vi "ObjectFactory.vi"(0 "GOject":refnum<vi>, 5 "error in (no error)":errorcluster) -> (14 "Object":refnum<class "Object.lvclass">, 15 "Is Indicator":bool, 16 "Is Control":bool, 17 "Is Visible":bool, 19 "error out":errorcluster)   [LabVIEW 2014, in "FrontPanelPublisher.lvlib" / "WebFrontPanel.lvclass"]
doc: "Convert FP refs into \"HTML\" objects"
uses:
  WebFrontPanel.lvclass
  Object_class/Object.lvclass
  Object_class/Attributes.ctl
  Object_class/Coordinates.ctl
  Control_class/Attributes.ctl
  Text_class/Text.lvclass
  BooleanControl_class/Attributes.ctl
  Numeric_class/Attributes.ctl
  String_class/Attributes.ctl
  Graph_class/Attributes.ctl
  Select_class/Attributes.ctl
  Progressbar_class/Attributes.ctl
  Text_class/Attributes.ctl
  Control_class/Control.lvclass
  BooleanControl_class/BooleanControl.lvclass
  Graph_class/Graph.lvclass
  Numeric_class/Numeric.lvclass
  FrontPanelPublisher.lvlib
  String_class/String.lvclass
  Select_class/Select.lvclass
  Progressbar_class/Progressbar.lvclass
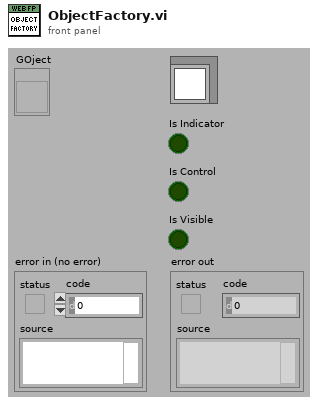
[diagram p1: front panel]
types:
  T1 = typedef "FrontPanelPublisher.lvlib/Object.lvclass/Attributes.ctl" = cluster{"UID":i32, "Type":string, "Coordinates":T2, "Reference":refnum<vi>}
  T2 = typedef "FrontPanelPublisher.lvlib/Object.lvclass/Coordinates.ctl" = cluster{"Left":i32, "Top":i32, "Height":u32, "Width":u32}
  T3 = typedef "FrontPanelPublisher.lvlib/Control.lvclass/Attributes.ctl" = cluster{"Description":string, "Indicator":bool, "Default Value":variant, "Control Index":i32, "Label":refnum<class "Text.lvclass">, "Caption":refnum<class "Text.lvclass">, "Use Picture":bool, "Image1 b64":string, "Image2 b64":string}
  T4 = typedef "FrontPanelPublisher.lvlib/BooleanControl.lvclass/Attributes.ctl" = cluster{"Boolean ref":refnum<vi>, "Switching":bool, "Boolean Strings":string[], "Text":refnum<class "Text.lvclass">}
  T5 = typedef "FrontPanelPublisher.lvlib/Numeric.lvclass/Attributes.ctl" = cluster{"unused":dbl}
  T6 = typedef "FrontPanelPublisher.lvlib/String.lvclass/Attributes.ctl" = cluster{"unused":string}
  T7 = typedef "FrontPanelPublisher.lvlib/Graph.lvclass/Attributes.ctl" = cluster{"not used":dbl}
  T8 = typedef "FrontPanelPublisher.lvlib/Select.lvclass/Attributes.ctl" = cluster{"not used":dbl}
  T9 = typedef "FrontPanelPublisher.lvlib/Progressbar.lvclass/Attributes.ctl" = cluster{"not used":dbl}
  T10 = cluster{"Object":T1, "Control":T3, "Boolean":T4, "Numeric":T5, "String":T6, "Graph":T7, "Select":T8, "Progressbar":T9, "Object out":refnum<class "Object.lvclass">, "Label":refnum<class "Text.lvclass">, "Caption":refnum<class "Text.lvclass">, "Is Indicator":bool, "Is Control":bool, "Is Visible":bool}
  T11 = typedef "FrontPanelPublisher.lvlib/Text.lvclass/Attributes.ctl" = cluster{"Text":string, "Font":string, "Font Size":u32, "Visible":bool}
  T12 = typedef "LVRectTypeDef.ctl" = cluster{"Left":i16, "Top":i16, "Right":i16, "Bottom":i16}
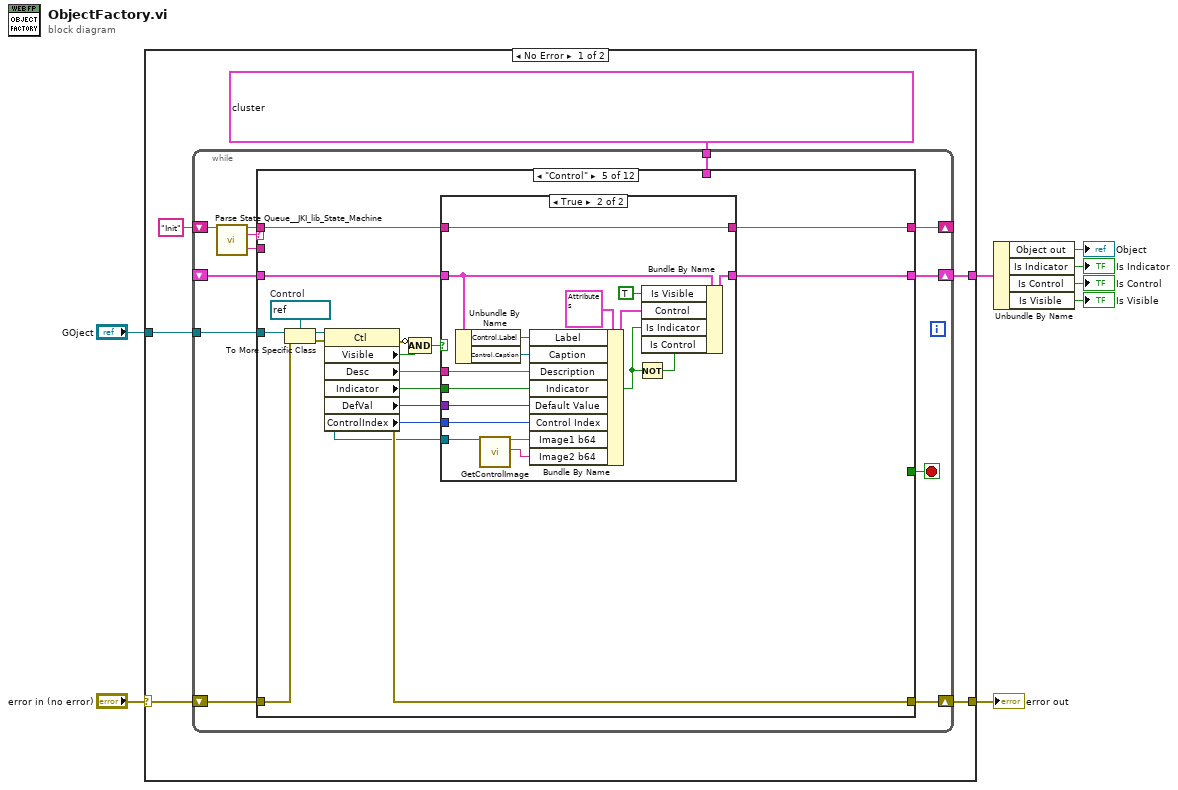
[diagram p0: block diagram]
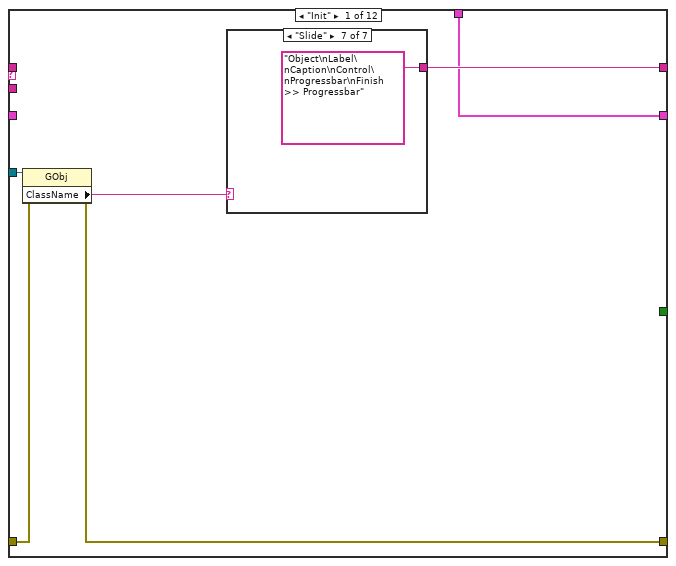
[diagram p2: hidden frame]
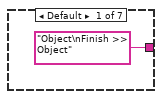
[diagram p3: hidden frame]
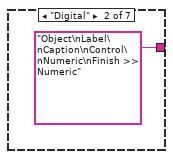
[diagram p4: hidden frame]
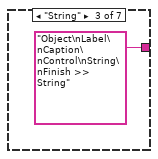
[diagram p5: hidden frame]
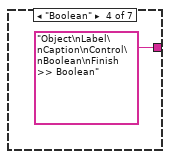
[diagram p6: hidden frame]
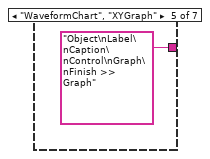
[diagram p7: hidden frame]
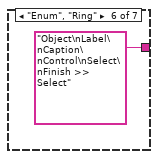
[diagram p8: hidden frame]
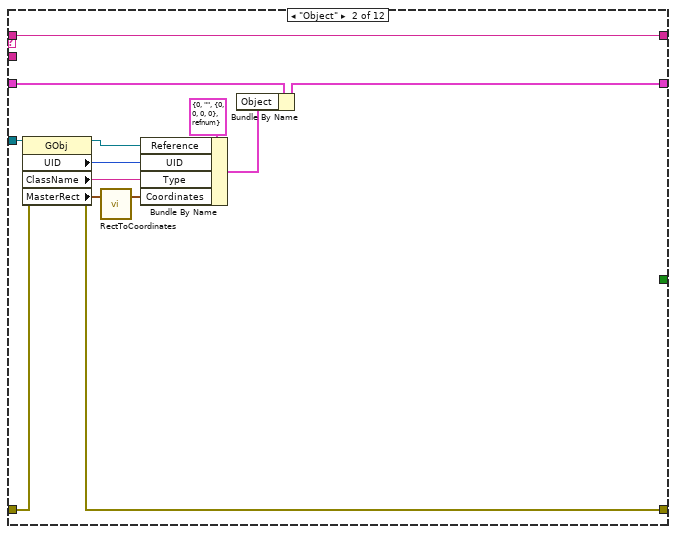
[diagram p9: hidden frame]
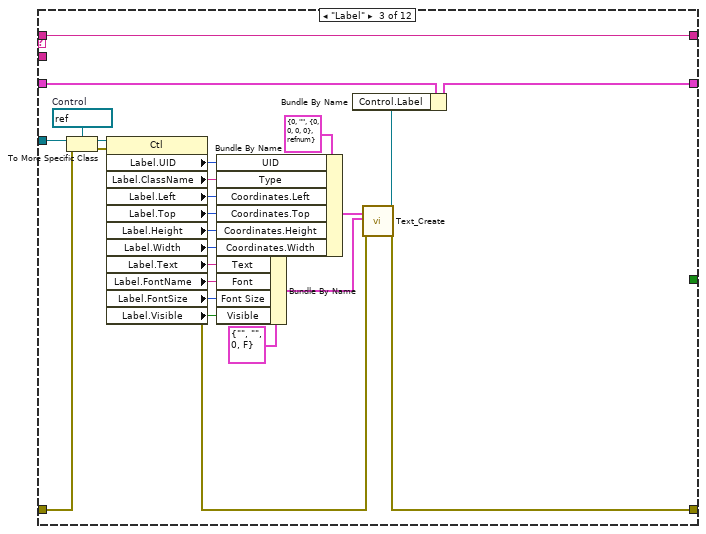
[diagram p10: hidden frame]
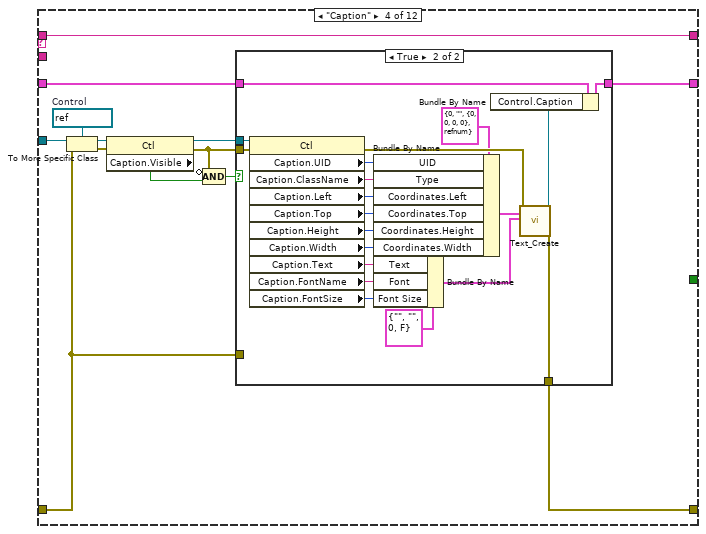
[diagram p11: hidden frame]
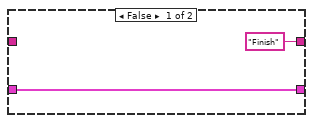
[diagram p13: hidden frame]
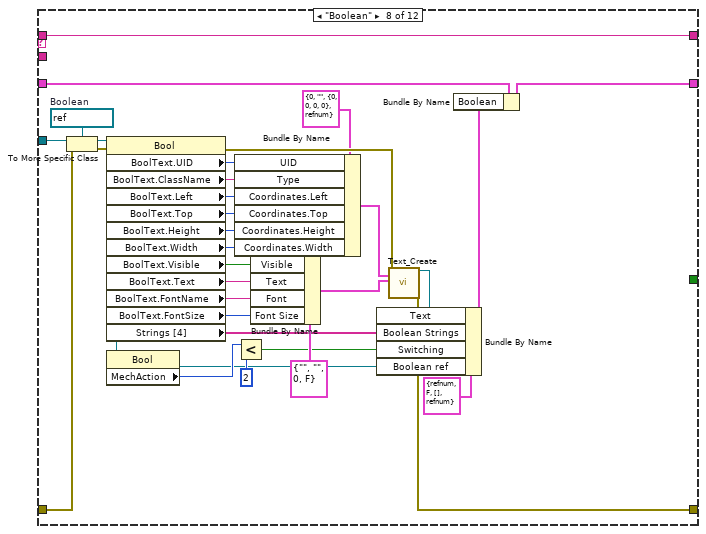
[diagram p16: hidden frame]
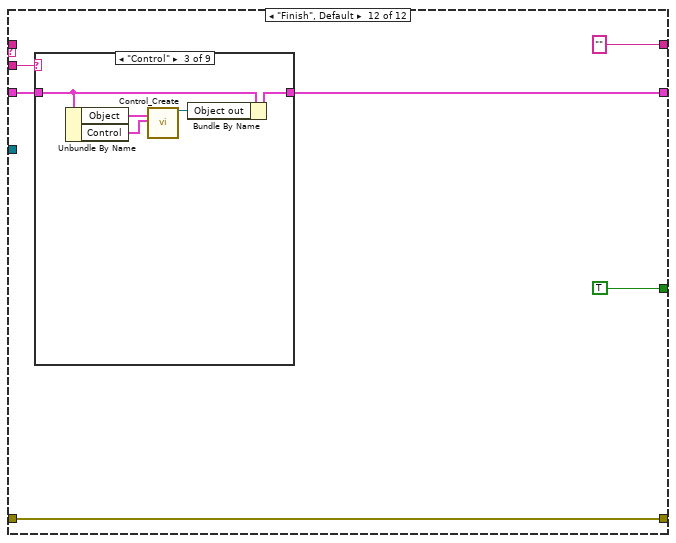
[diagram p20: hidden frame]
diagram:
  n1 = case shown="No Error" "error in (no error)" {
    selector: "error in (no error)" -> [w13 w245]
    tunnel: [w14 w245] -> w7
    tunnel: "GOject" -> [w12 _]
    tunnel: [w9 _] -> w5
    frame No Error {
      n2 = while {
        tunnel: w12 -> [w24]
        shift-right: [w15] -> _
        shift-left: "Init" -> [w19]
        shift-right: [w23] -> w9
        shift-left: _ -> [w22]
        shift-right: [w25] -> w14
        shift-left: w13 -> [w26]
        tunnel: T10 {"Object"={"UID"=0, "Type"="", "Coordinates"={"Left"=0, "Top"=0, "Height"=0, "Width"=0}, "Reference"=refnum}, "Control"={"Description"="", "Indicator"=FALSE, "Default Value"=variant, "Control Index"=0, "Label"=refnum, "Caption"=refnum, "Use Picture"=FALSE, "Image1 b64"="", "Image2 b64"=""}, "Boolean"={"Boolean ref"=refnum, "Switching"=FALSE, "Boolean Strings"=[], "Text"=refnum}, "Numeric"={"unused"=0.0}, "String"={"unused"=""}, "Graph"={"not used"=0.0}, "Select"={"not used"=0.0}, "Progressbar"={"not used"=0.0}, "Object out"=refnum, "Label"=refnum, "Caption"=refnum, "Is Indicator"=FALSE, "Is Control"=FALSE, "Is Visible"=FALSE} -> [w21]
        stop <- w20 stop-if-true
        n3 = call <vilib>:"Parse State Queue__JKI_lib_State_Machine.vi"("State Queue"=w19) -> ("Remaining States"=w16:string, "Current State"=w18:string, "Arguments"=w17:string)  [unwired: 12 in]
        n4 = case shown="\"Control\"" w18 {
          tunnel: w24 -> [w30 w48 w72 w84 w124 _ _ w180 _ _ _ _]
          tunnel: [w28 w45 w60 w79 w115 w149 w152 w177 w186 w189 w192 ""] -> w15
          tunnel: [w27 w47 w61 w80 w118 w148 w151 w178 w184 w187 w190 w194] -> w23
          tunnel: w22 -> [_ w46 w62 w81 w123 w148 w151 w179 w184 w187 w190 w193]
          tunnel: [w31 w51 w75 w88 w126 w147 w150 w183 w185 w188 w191 w198] -> w25
          tunnel: w26 -> [w32 w52 w76 w87 w127 w147 w150 w182 w185 w188 w191 w198]
          tunnel: w21 -> [w27 _ _ _ _ _ _ _ _ _ _ _]
          tunnel: [_ _ _ _ _ _ _ _ _ _ _ TRUE] -> w20
          tunnel: w17 -> [_ _ _ _ _ _ _ _ _ _ _ w195]
          tunnel: w16 -> [_ w45 w60 w79 w114 w149 w152 w177 w186 w189 w192 _]
          frame "Init" {
            n5 = property class="GObj"(reference=w30, error in=w32) -> (error out=w31:errorcluster, "ClassName"=w29:string)  [unwired: 1 out]
            n6 = case shown="\"Slide\"" w29 {
              tunnel: ["Object\nFinish >> Object" "Object\nLabel\nCaption\nControl\nNumeric\nFinish >> Numeric" "Object\nLabel\nCaption\nControl\nString\nFinish >> String" "Object\nLabel\nCaption\nControl\nBoolean\nFinish >> Boolean" "Object\nLabel\nCaption\nControl\nGraph\nFinish >> Graph" "Object\nLabel\nCaption\nControl\nSelect\nFinish >> Select" "Object\nLabel\nCaption\nControl\nProgressbar\nFinish >> Progressbar"] -> w28
              frame Default {
              }
              frame "Digital" {
              }
              frame "String" {
              }
              frame "Boolean" {
              }
              frame "WaveformChart", "XYGraph" {
              }
              frame "Enum", "Ring" {
              }
              frame "Slide" {
              }
            }
          }
          frame "Object" {
            n7 = property class="GObj"(reference=w48, error in=w52) -> (reference out=w40:refnum<vi>, error out=w51:errorcluster, "UID"=w49:i32, "ClassName"=w50:string, "MasterRect"=w42:T12)
            n8 = call "RectToCoordinates.vi"("Rect"=w42) -> ("Coordinates"=w41:T2)  [unwired: 2 in]
            n9 = Bundle By Name(cluster=T1 {"UID"=0, "Type"="", "Coordinates"={"Left"=0, "Top"=0, "Height"=0, "Width"=0}, "Reference"=refnum} ("Object Attributes"), "Reference"=w40, "UID"=w49, "Type"=w50, "Coordinates"=w41) -> (w43:T1)
            n10 = Bundle By Name(cluster=w46, "Object"=w43) -> (w47:T10)
          }
          frame "Label" {
            w74 = refnum<vi> refnum  # Control
            n11 = To More Specific Class(target class=w74, reference=w72, error in=w76) -> (specific class reference=w73:refnum<vi>, error out=w77:errorcluster)
            n12 = property class="Ctl"(reference=w73, error in=w77) -> (error out=w54:errorcluster, "Label.UID"=w71:i32, "Label.ClassName"=w70:string, "Label.Left"=w69:i32, "Label.Top"=w68:i32, "Label.Height"=w67:u32, "Label.Width"=w66:u32, "Label.Text"=w65:string, "Label.FontName"=w64:string, "Label.FontSize"=w63:u32, "Label.Visible"=w53:bool)  [unwired: 1 out]
            n13 = Bundle By Name(cluster=T1 {"UID"=0, "Type"="", "Coordinates"={"Left"=0, "Top"=0, "Height"=0, "Width"=0}, "Reference"=refnum} ("Object Attributes"), "UID"=w71, "Type"=w70, "Coordinates.Left"=w69, "Coordinates.Top"=w68, "Coordinates.Height"=w67, "Coordinates.Width"=w66) -> (w57:T1)
            n14 = Bundle By Name(cluster=T11 {"Text"="", "Font"="", "Font Size"=0, "Visible"=FALSE} ("Text Attributes"), "Text"=w65, "Font"=w64, "Font Size"=w63, "Visible"=w53) -> (w56:T11)
            n15 = call "Text_Create.vi"("Object Attributes"=w57, "Text Attributes"=w56, "error in (no error)"=w54) -> ("reference out"=w55:refnum<class "Text.lvclass">, "error out"=w75:errorcluster)  [unwired: 15 in]
            n16 = Bundle By Name(cluster=w62, "Control.Label"=w55) -> (w61:T10)
          }
          frame "Caption" {
            w86 = refnum<vi> refnum  # Control
            n17 = To More Specific Class(target class=w86, reference=w84, error in=w87) -> (specific class reference=w85:refnum<vi>, error out=w90:errorcluster)
            n18 = property class="Ctl"(reference=w85, error in=w90) -> (reference out=w78:refnum<vi>, error out=w89:errorcluster, "Caption.Visible"=w83:bool)
            n19 = Compound Arithmetic op=AND(invert w89, w83) -> (w82:bool)
            n20 = case shown="True" w82 {
              tunnel: w81 -> [w91 w105]
              tunnel: [w91 w104] -> w80
              tunnel: w78 -> [_ w102]
              tunnel: w89 -> [_ w112]
              tunnel: [w92 w110] -> w88
              tunnel: w87 -> [w92 _]
              frame False {
              }
              frame True {
                n21 = property class="Ctl"(reference=w102, error in=w112) -> (error out=w111:errorcluster, "Caption.UID"=w101:i32, "Caption.ClassName"=w100:string, "Caption.Left"=w99:i32, "Caption.Top"=w98:i32, "Caption.Height"=w97:u32, "Caption.Width"=w96:u32, "Caption.Text"=w95:string, "Caption.FontName"=w94:string, "Caption.FontSize"=w93:u32)  [unwired: 1 out]
                n22 = Bundle By Name(cluster=T1 {"UID"=0, "Type"="", "Coordinates"={"Left"=0, "Top"=0, "Height"=0, "Width"=0}, "Reference"=refnum} ("Object Attributes"), "UID"=w101, "Type"=w100, "Coordinates.Left"=w99, "Coordinates.Top"=w98, "Coordinates.Height"=w97, "Coordinates.Width"=w96) -> (w107:T1)
                n23 = Bundle By Name(cluster=T11 {"Text"="", "Font"="", "Font Size"=0, "Visible"=FALSE} ("Text Attributes"), "Text"=w95, "Font"=w94, "Font Size"=w93) -> (w106:T11)
                n24 = call "Text_Create.vi"("Object Attributes"=w107, "Text Attributes"=w106, "error in (no error)"=w111) -> ("reference out"=w103:refnum<class "Text.lvclass">, "error out"=w110:errorcluster)  [unwired: 15 in]
                n25 = Bundle By Name(cluster=w105, "Control.Caption"=w103) -> (w104:T10)
              }
            }
          }
          frame "Control" {
            w125 = refnum<vi> refnum  # Control
            n26 = To More Specific Class(target class=w125, reference=w124, error in=w127) -> (specific class reference=w113:refnum<vi>, error out=w128:errorcluster)
            n27 = property class="Ctl"(reference=w113, error in=w128) -> (error out=w126:errorcluster, "Visible"=w116:bool, "Desc"=w122:string, "Indicator"=w121:bool, "DefVal"=w120:variant, "ControlIndex"=w119:i32)  [unwired: 1 out]
            n28 = Compound Arithmetic op=AND(invert w126, w116) -> (w117:bool)
            n29 = case shown="True" w117 {
              tunnel: w123 -> [w130 w140]
              tunnel: w122 -> [_ w146]
              tunnel: w121 -> [_ w136]
              tunnel: w120 -> [_ w145]
              tunnel: w119 -> [_ w144]
              tunnel: [w130 w131] -> w118
              tunnel: ["Finish" w141] -> w115
              tunnel: w114 -> [_ w141]
              tunnel: w113 -> [_ w132]
              frame False {
              }
              frame True {
                n30 = Unbundle By Name(w140) -> ("Control.Label"=w139:refnum<class "Text.lvclass">, "Control.Caption"=w138:refnum<class "Text.lvclass">)
                n31 = call "GetControlImage.vi"("Control ref"=w132) -> ("base64 encoded <img> string 1"=w134:string, "base64 encoded <img> string 2"=w133:string)  [unwired: 16 in, 1 out]
                n32 = Bundle By Name(cluster=T3 {"Description"="", "Indicator"=FALSE, "Default Value"=variant, "Control Index"=0, "Label"=refnum, "Caption"=refnum, "Use Picture"=FALSE, "Image1 b64"="", "Image2 b64"=""} ("Control Attributes"), "Label"=w139, "Caption"=w138, "Description"=w146, "Indicator"=w136, "Default Value"=w145, "Control Index"=w144, "Image1 b64"=w134, "Image2 b64"=w133) -> (w142:T3)
                n33 = Not(x=w136) -> (.not. x?=w135:bool)
                n34 = Bundle By Name(cluster=w140, "Is Visible"=TRUE, "Control"=w142, "Is Indicator"=w136, "Is Control"=w135) -> (w131:T10)
              }
            }
          }
          frame "Numeric" {
            # "All properties are queried at run time"
          }
          frame "String" {
            # "All properties are queried at run time"
          }
          frame "Boolean" {
            w181 = refnum<vi> refnum  # Boolean
            n35 = To More Specific Class(target class=w181, reference=w180, error in=w182) -> (specific class reference=w153:refnum<vi>, error out=w155:errorcluster)
            n36 = property class="Bool"(reference=w153, error in=w155) -> (error out=w176:errorcluster, "BoolText.UID"=w166:i32, "BoolText.ClassName"=w165:string, "BoolText.Left"=w164:i32, "BoolText.Top"=w163:i32, "BoolText.Height"=w162:u32, "BoolText.Width"=w161:u32, "BoolText.Visible"=w156:bool, "BoolText.Text"=w160:string, "BoolText.FontName"=w159:string, "BoolText.FontSize"=w158:u32, "Strings [4]"=w157:string[])  [unwired: 1 out]
            n37 = property class="Bool"(reference=w153) -> ("MechAction"=w154:u32)  [unwired: 1 in, 2 out]
            n38 = Bundle By Name(cluster=T1 {"UID"=0, "Type"="", "Coordinates"={"Left"=0, "Top"=0, "Height"=0, "Width"=0}, "Reference"=refnum} ("Object Attributes"), "UID"=w166, "Type"=w165, "Coordinates.Left"=w164, "Coordinates.Top"=w163, "Coordinates.Height"=w162, "Coordinates.Width"=w161) -> (w171:T1)
            n39 = Less?(x=w154, y=u32 2) -> (x < y?=w167:bool)
            n40 = Bundle By Name(cluster=T11 {"Text"="", "Font"="", "Font Size"=0, "Visible"=FALSE} ("Text Attributes"), "Visible"=w156, "Text"=w160, "Font"=w159, "Font Size"=w158) -> (w170:T11)
            n41 = call "Text_Create.vi"("Object Attributes"=w171, "Text Attributes"=w170, "error in (no error)"=w176) -> ("reference out"=w169:refnum<class "Text.lvclass">, "error out"=w183:errorcluster)  [unwired: 15 in]
            n42 = Bundle By Name(cluster=T4 {"Boolean ref"=refnum, "Switching"=FALSE, "Boolean Strings"=[], "Text"=refnum} ("BooleanControl Attributes"), "Text"=w169, "Boolean Strings"=w157, "Switching"=w167, "Boolean ref"=w153) -> (w168:T4)
            n43 = Bundle By Name(cluster=w179, "Boolean"=w168) -> (w178:T10)
          }
          frame "Graph" {
            # "All properties are queried at run time"
          }
          frame "Select" {
            # "All properties are queried at run time"
          }
          frame "Progressbar" {
            # "All properties are queried at run time"
          }
          frame "Finish", Default {
            n44 = case shown="\"Control\"" w195 {
              tunnel: [w199 w201 w207 w210 w218 w224 w230 w236 w242] -> w194
              tunnel: w193 -> [w199 w203 w208 w214 w220 w226 w232 w238 w244]
              frame Default {
              }
              frame "Object" {
                n45 = Unbundle By Name(w203) -> ("Object"=w202:T1)
                n46 = call "Object_Create.vi"("Object Attributes"=w202) -> ("reference out"=w200:refnum<class "Object.lvclass">)  [unwired: 17 in, 1 out]
                n47 = Bundle By Name(cluster=w203, "Object out"=w200) -> (w201:T10)
              }
              frame "Control" {
                n48 = Unbundle By Name(w208) -> ("Object"=w205:T1, "Control"=w204:T3)
                n49 = call "Control_Create.vi"("Object Attributes"=w205, "Control Attributes"=w204) -> ("reference out"=w206:refnum<class "Control.lvclass">)  [unwired: 16 in, 1 out]
                n50 = Bundle By Name(cluster=w208, "Object out"=w206) -> (w207:T10)
              }
              frame "Boolean" {
                n51 = Unbundle By Name(w214) -> ("Object"=w213:T1, "Control"=w212:T3, "Boolean"=w211:T4)
                n52 = call "BooleanControl_Create.vi"("Object Attributes"=w213, "Control Attributes"=w212, "BooleanControl Attributes"=w211) -> ("reference out"=w209:refnum<class "BooleanControl.lvclass">)  [unwired: 15 in, 1 out]
                n53 = Bundle By Name(cluster=w214, "Object out"=w209) -> (w210:T10)
              }
              frame "Graph" {
                n54 = Unbundle By Name(w220) -> ("Object"=w216:T1, "Control"=w219:T3, "Graph"=w215:T7)
                n55 = call "Graph_Create.vi"("Object Attributes"=w216, "Control Attributes"=w219, "Graph Attributes"=w215) -> ("reference out"=w217:refnum<class "Graph.lvclass">)  [unwired: 15 in, 1 out]
                n56 = Bundle By Name(cluster=w220, "Object out"=w217) -> (w218:T10)
              }
              frame "Numeric" {
                n57 = Unbundle By Name(w226) -> ("Object"=w222:T1, "Control"=w225:T3, "Numeric"=w221:T5)
                n58 = call "Numeric_Create.vi"("Object Attributes"=w222, "Control Attributes"=w225, "Graph Attributes"=w221) -> ("reference out"=w223:refnum<class "Numeric.lvclass">)  [unwired: 15 in, 1 out]
                n59 = Bundle By Name(cluster=w226, "Object out"=w223) -> (w224:T10)
              }
              frame "String" {
                n60 = Unbundle By Name(w232) -> ("Object"=w228:T1, "Control"=w231:T3, "String"=w227:T6)
                n61 = call "String_Create.vi"("Object Attributes"=w228, "Control Attributes"=w231, "String Attributes"=w227) -> ("reference out"=w229:refnum<class "String.lvclass">)  [unwired: 15 in, 1 out]
                n62 = Bundle By Name(cluster=w232, "Object out"=w229) -> (w230:T10)
              }
              frame "Select" {
                n63 = Unbundle By Name(w238) -> ("Object"=w234:T1, "Control"=w237:T3, "Select"=w233:T8)
                n64 = call "Select_Create.vi"("Object Attributes"=w234, "Control Attributes"=w237, "Select Attributes"=w233) -> ("reference out"=w235:refnum<class "Select.lvclass">)  [unwired: 15 in, 1 out]
                n65 = Bundle By Name(cluster=w238, "Object out"=w235) -> (w236:T10)
              }
              frame "Progressbar" {
                n66 = Unbundle By Name(w244) -> ("Object"=w240:T1, "Control"=w243:T3, "Progressbar"=w239:T9)
                n67 = call "Progressbar_Create.vi"("Object Attributes"=w240, "Control Attributes"=w243, "Progressbar Attributes"=w239) -> ("reference out"=w241:refnum<class "Progressbar.lvclass">)  [unwired: 15 in, 1 out]
                n68 = Bundle By Name(cluster=w244, "Object out"=w241) -> (w242:T10)
              }
            }
          }
        }
      }
    }
    frame Error {
    }
  }
  "error out" <- w7
  n69 = Unbundle By Name(w5) -> ("Object out"=→"Object":refnum<class "Object.lvclass">, "Is Indicator"=→"Is Indicator":bool, "Is Control"=→"Is Control":bool, "Is Visible"=→"Is Visible":bool)
